vi "overlay_crossmarks.vi"(6 "Color":u32, 8 "error in (no error)":errorcluster, 9 "Width":u32=2, 10 "Box Rectangle":T2, 11 "Refnum in":T1) -> (0 "error out":errorcluster, 3 "Refnum out":T1)   [LabVIEW 2019]
uses:
  <vilib>/vision/Image Controls.llb/IMAQ Image.ctl
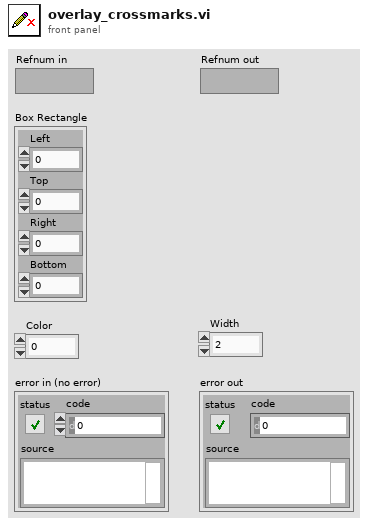
[diagram p1: front panel]
types:
  T1 = typedef "IMAQ Image.ctl" = refnum<image>
  T2 = cluster{"Left":i32, "Top":i32, "Right":i32, "Bottom":i32}
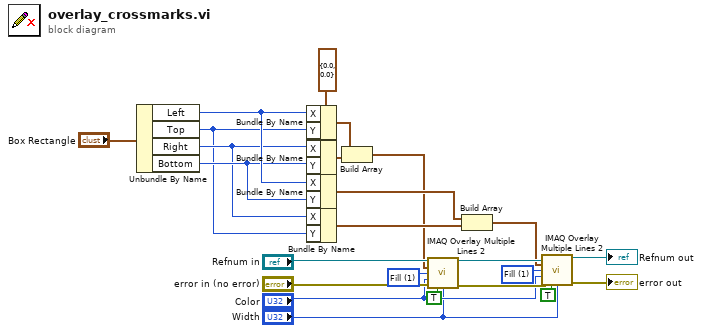
[diagram p0: block diagram]
diagram:
  w13 = u32 1 items=["Frame", "Fill"] ("Drawing Mode (Frame)")
  w20 = cluster{"X":dbl, "Y":dbl} {"X"=0.0, "Y"=0.0} ("Point Coordinates")
  w24 = u32 1 items=["Frame", "Fill"] ("Drawing Mode (Frame)")
  n1 = Unbundle By Name("Box Rectangle") -> ("Left"=w19:i32, "Top"=w1:i32, "Right"=w2:i32, "Bottom"=w18:i32)
  n2 = Bundle By Name(cluster=w20, "X"=w19, "Y"=w1) -> (w17:cluster{"X":dbl, "Y":dbl})
  n3 = Bundle By Name(cluster=w20, "X"=w2, "Y"=w18) -> (w16:cluster{"X":dbl, "Y":dbl})
  n4 = Bundle By Name(cluster=w20, "X"=w19, "Y"=w18) -> (w14:cluster{"X":dbl, "Y":dbl})
  n5 = Bundle By Name(cluster=w20, "X"=w2, "Y"=w1) -> (w15:cluster{"X":dbl, "Y":dbl})
  n6 = Build Array(w17, w16) -> (w7:cluster{"X":dbl, "Y":dbl}[])
  n7 = call "IMAQ Overlay Multiple Lines 2"("Image"="Refnum in", "Line End Points"=w7, "Drawing Mode (Frame)"=w24, "Color"="Color", "error in (no error)"="error in (no error)", "Maintain Width?"=TRUE, "Width"="Width") -> ("Image Out"=w11:T1, "error out"=w12:errorcluster)  [unwired: 7 in]
  n8 = Build Array(w14, w15) -> (w8:cluster{"X":dbl, "Y":dbl}[])
  n9 = call "IMAQ Overlay Multiple Lines 2"("Image"=w11, "Line End Points"=w8, "Drawing Mode (Frame)"=w13, "Color"="Color", "error in (no error)"=w12, "Maintain Width?"=TRUE, "Width"="Width") -> ("Image Out"=→"Refnum out":T1, "error out"=→"error out":errorcluster)  [unwired: 7 in]
